vi "Return ID to Pool.vi"(8 "error in (no error)":errorcluster, 9 "timeout in ms (0)":i32 format="%d ms", 10 "id":i32, 11 "ID Pool in":refnum<class "ID Pool.lvclass">) -> (0 "error out":errorcluster, 1 "timed out?":bool, 3 "ID Pool out":refnum<class "ID Pool.lvclass">)   [LabVIEW 2017, in "DSF Core.lvlib" / "ID Pool.lvclass"]
uses:
  ID Pool.lvclass
  C:/Git/DSF/Data Sharing Framework/Source/Core/Engine/Classes/Thread Pool/Pool.lvclass
  Pool.lvclass/Pool.ctl
  Return ID Timeout.vi
  Pool.lvclass
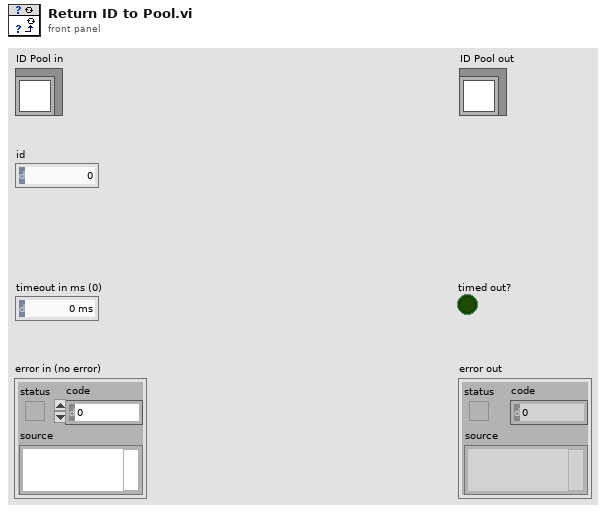
[diagram p1: front panel]
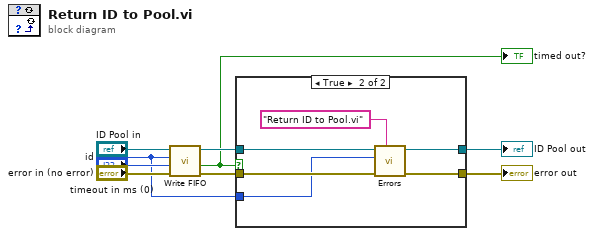
[diagram p0: block diagram]
diagram:
  n1 = call "Write FIFO.vi"("error in (no error)"="error in (no error)", "timeout in ms (0)"="timeout in ms (0)", "element"="id", "Pool in"="ID Pool in") -> ("error out"=w5:errorcluster, "timed out?"=w4:bool, "Pool out"=w6:refnum<class "ID Pool.lvclass">)  [unwired: 5 in]
  "timed out?" <- w4
  n2 = case shown="True" w4 {
    tunnel: w6 -> [w11 w17]
    tunnel: w5 -> [w10 w16]
    tunnel: [w11 w15] -> w3
    tunnel: [w10 w14] -> w2
    tunnel: "id" -> [_ w12]
    frame False {
    }
    frame True {
      n3 = call-poly "Errors.vi"("error source vi name"="Return ID to Pool.vi", "error in (no error)"=w16, "id"=w12, "ID Pool in"=w17) -> ("error out"=w14:errorcluster, "ID Pool out"=w15:refnum<class "ID Pool.lvclass">)  [unwired: 6 in]
    }
  }
  "error out" <- w2
  "ID Pool out" <- w3
